vi "Run_2_of_5_Tests.vi"() -> ()   [LabVIEW 2019]
panel:
  out "Matrix":bool
  out "PID":bool
  out "Math Utils":bool
  out "Linear Filter":bool
  out "Linear System Loop":bool
  out "All Tests Finished":bool
  out "Holonomic Drive Ctrl":bool
  out "Linear Plant Inv FF":bool
  out "Numerical Jacobian":bool
  out "Merwe Scaled Sigma Pts":bool
  out "Numerical Integration":bool
  out "Median Filter":bool
  out "Linear System ID":bool
  out "Kalman filter":bool
  out "PID Input / Output":bool
  out "Linear Quadradtic Regulator":bool
  # "FORMAL TRAJECTORY / CONTROL LIBRARY TEST PROCEDURE"
  # "FUNCTION NOT\nIMPLEMENTED"
  # "Extended Kalman Filter"
  # "Mech Drive Kinematics"
  # "Mech Drive Odometry"
  # "Mech Drive Pose Est"
  # "FUNCTION NOT\nIMPLEMENTED"
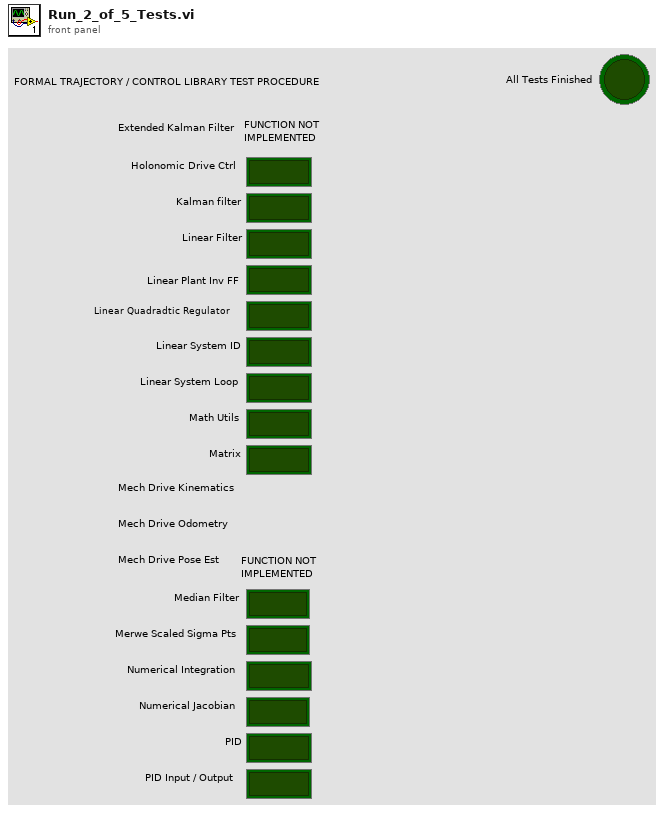
[diagram p1: front panel]
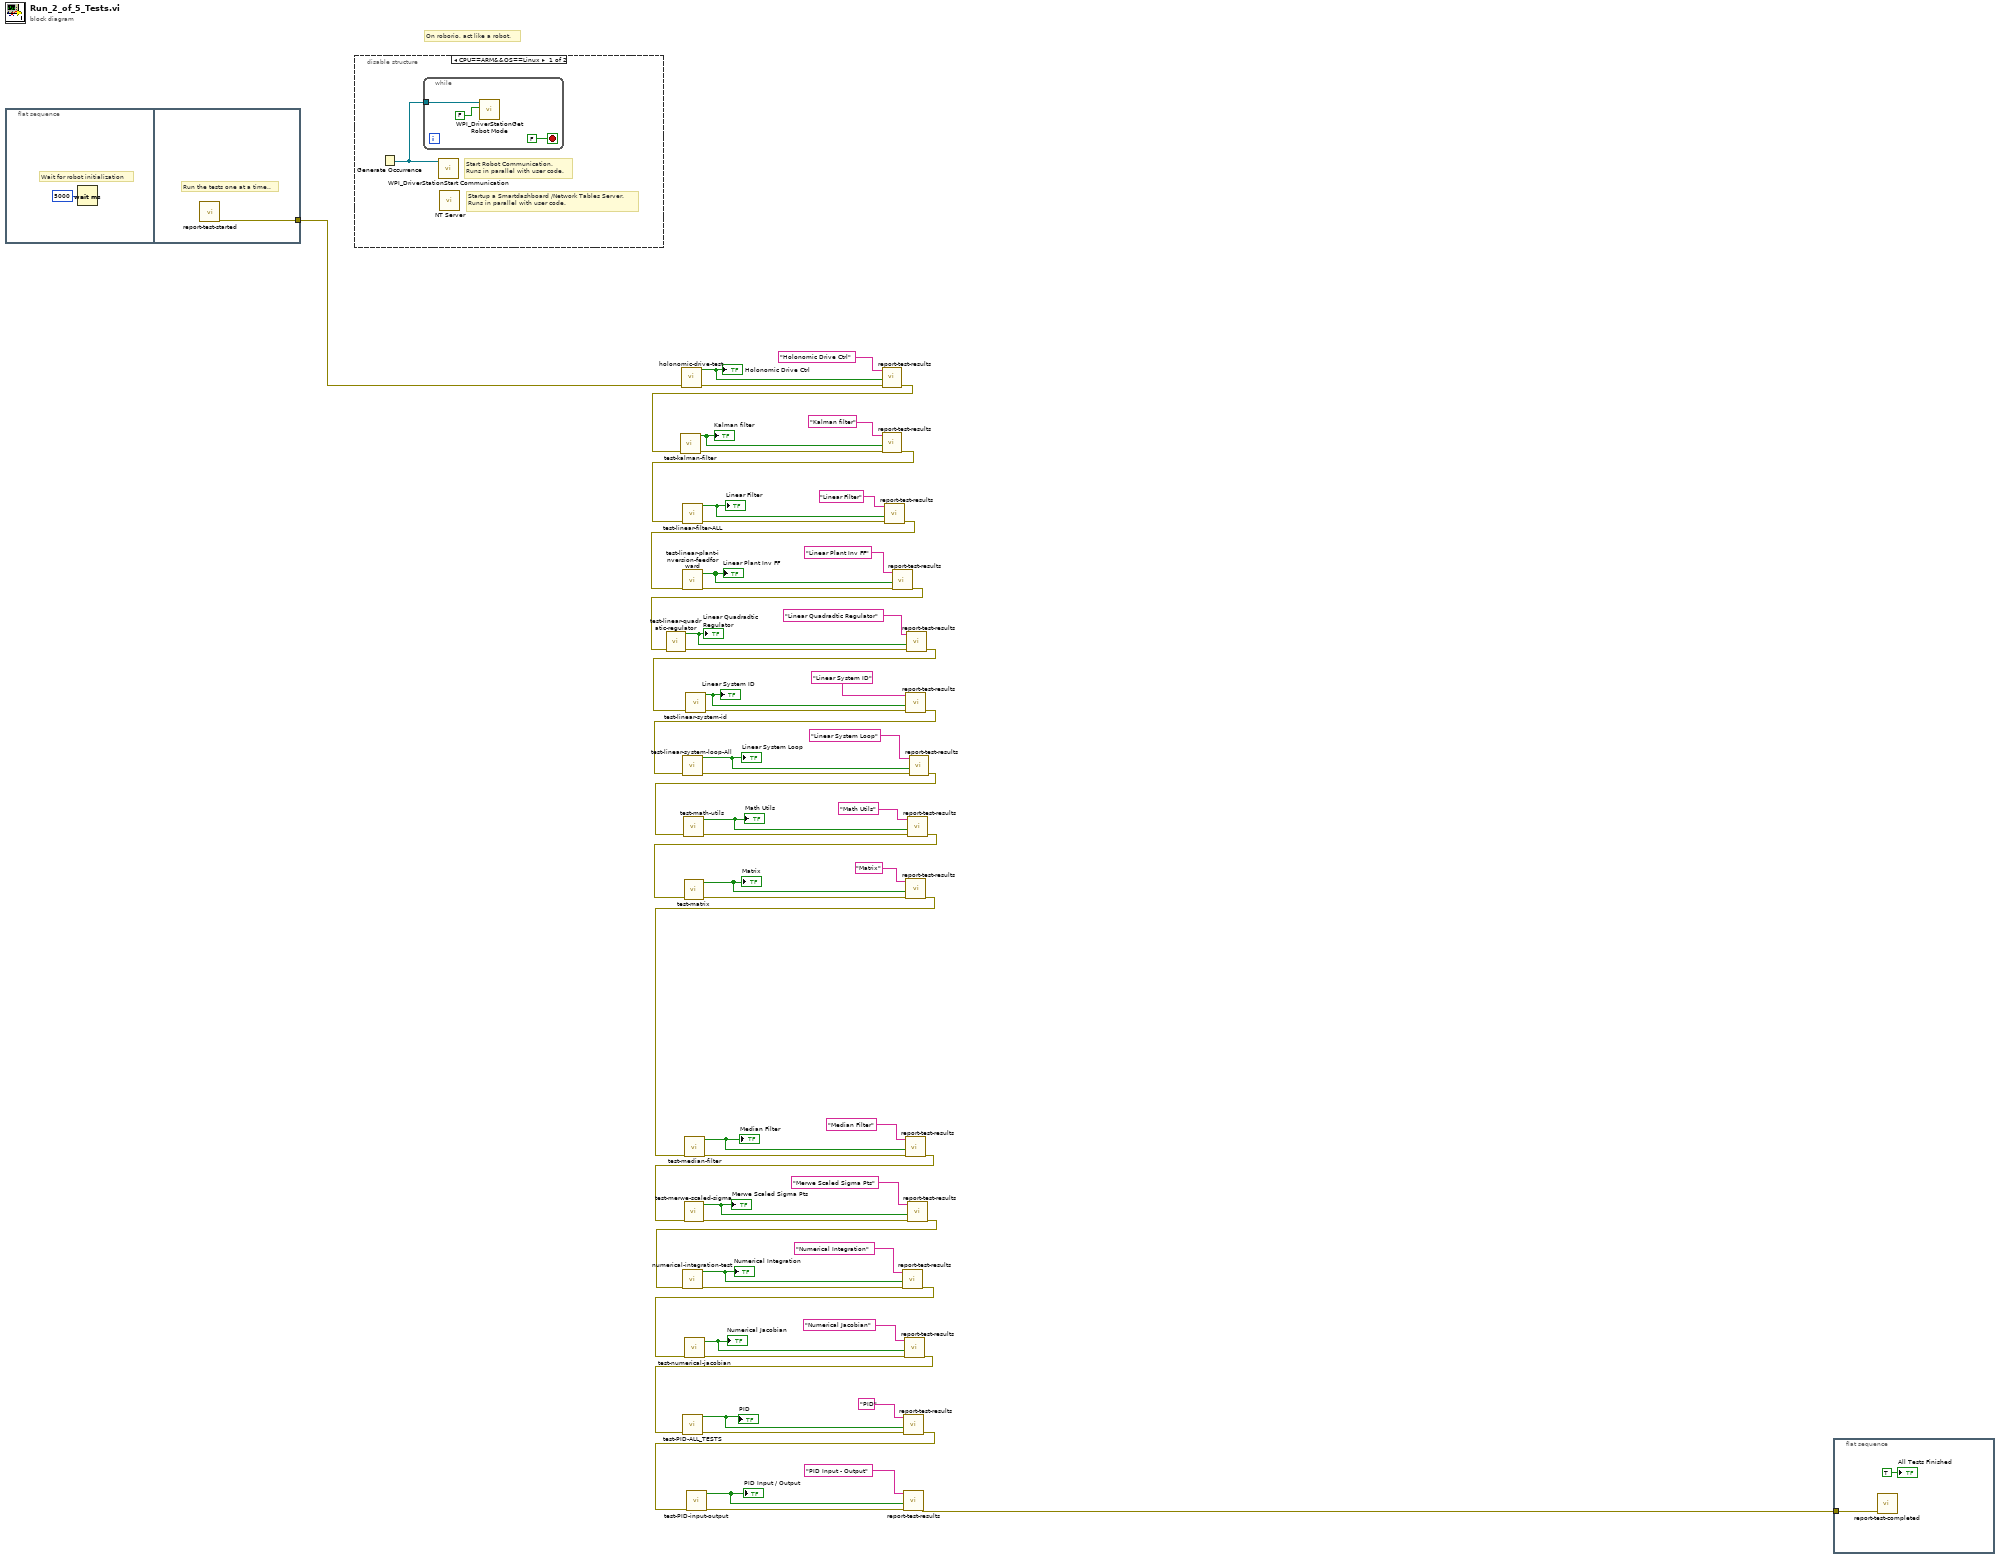
[diagram p0: block diagram]
diagram:
  # "On roborio, act like a robot."
  n1 = flat-sequence {
    tunnel: [w63] -> w1
    frame #0 {
      # "Wait for robot initialization"
      n2 = Wait (ms)(milliseconds to wait=u32 5000) -> ()  [unwired: 1 out]
    }
    frame #1 {
      # "Run the tests one at a time.."
      n3 = call "report-test-started.vi"() -> ("error out"=w63:errorcluster)  [unwired: 11 in]
    }
  }
  n4 = disable-structure shown="CPU==ARM&&OS==Linux" {
    frame condition #0 (active) {
      # "Startup a Smartdashboard /Network Tables Server.\nRuns in parallel with user code."
      # "Start Robot Communication.\nRuns in parallel with user code."
      n5 = Generate Occurrence() -> (w64:refnum<k4>)
      n6 = while {
        tunnel: w64 -> [w67]
        stop <- FALSE stop-if-true
        n7 = call <vilib>:"WPI_DriverStationGet Robot Mode.vi"("Finish"=FALSE, "DS Occurrence"=w67) -> ()  [unwired: 10 out]
      }
      n8 = call <vilib>:"WPI_DriverStationStart Communication.vi"("occurrence"=w64) -> ()  [unwired: 2 in, 9 out]
      n9 = call <vilib>:"NT Server.vi"() -> ()  [unwired: 12 in]
    }
    frame condition #1 {
    }
  }
  n10 = call "holonomic-drive-test.vi"("error in (no error)"=w1) -> ("error out"=w31:errorcluster, "ALL TESTS PASSED"=w59:bool)  [unwired: 9 in]
  "Holonomic Drive Ctrl" <- w59
  n11 = call "report-test-results.vi"("error in (no error)"=w31, "TestPassed"=w59, "Test Name"="Holonomic Drive Ctrl") -> ("error out"=w30:errorcluster)  [unwired: 8 in]
  n12 = call "test-kalman-filter.vi"("error in (no error)"=w30) -> ("error out"=w29:errorcluster, "ALL TESTS PASSED"=w58:bool)  [unwired: 9 in]
  "Kalman filter" <- w58
  n13 = call "report-test-results.vi"("error in (no error)"=w29, "TestPassed"=w58, "Test Name"="Kalman filter") -> ("error out"=w28:errorcluster)  [unwired: 8 in]
  n14 = call "test-linear-filter-ALL.vi"("error in (no error)"=w28) -> ("error out"=w26:errorcluster, "ALL TESTS GOOD"=w49:bool)  [unwired: 9 in]
  "Linear Filter" <- w49
  n15 = call "report-test-results.vi"("error in (no error)"=w26, "TestPassed"=w49, "Test Name"="Linear Filter") -> ("error out"=w25:errorcluster)  [unwired: 8 in]
  n16 = call "test-linear-plant-inversion-feedforward.vi"("error in (no error)"=w25) -> ("error out"=w24:errorcluster, "All Tests Passed"=w48:bool)  [unwired: 9 in]
  "Linear Plant Inv FF" <- w48
  n17 = call "report-test-results.vi"("error in (no error)"=w24, "TestPassed"=w48, "Test Name"="Linear Plant Inv FF") -> ("error out"=w23:errorcluster)  [unwired: 8 in]
  n18 = call "test-linear-quadratic-regulator.vi"("error in (no error)"=w23) -> ("error out"=w22:errorcluster, "ALL TESTS GOOD"=w47:bool)  [unwired: 9 in]
  "Linear Quadradtic Regulator" <- w47
  n19 = call "report-test-results.vi"("error in (no error)"=w22, "TestPassed"=w47, "Test Name"="Linear Quadradtic Regulator") -> ("error out"=w21:errorcluster)  [unwired: 8 in]
  n20 = call "test-linear-system-id.vi"("error in (no error)"=w21) -> ("error out"=w20:errorcluster, "All tests passed"=w46:bool)  [unwired: 9 in]
  "Linear System ID" <- w46
  n21 = call "report-test-results.vi"("error in (no error)"=w20, "TestPassed"=w46, "Test Name"="Linear System ID") -> ("error out"=w12:errorcluster)  [unwired: 8 in]
  n22 = call "test-linear-system-loop-All.vi"("error in (no error)"=w12) -> ("error out"=w13:errorcluster, "ALL TEsts Passed"=w45:bool)  [unwired: 9 in]
  "Linear System Loop" <- w45
  n23 = call "report-test-results.vi"("error in (no error)"=w13, "TestPassed"=w45, "Test Name"="Linear System Loop") -> ("error out"=w11:errorcluster)  [unwired: 8 in]
  n24 = call "test-math-utils.vi"("error in (no error)"=w11) -> ("error out"=w10:errorcluster, "ALL TESTS PASSED"=w44:bool)  [unwired: 9 in]
  "Math Utils" <- w44
  n25 = call "report-test-results.vi"("error in (no error)"=w10, "TestPassed"=w44, "Test Name"="Math Utils") -> ("error out"=w9:errorcluster)  [unwired: 8 in]
  n26 = call "test-matrix.vi"("error in (no error)"=w9) -> ("error out"=w14:errorcluster, "All Tests\nPassed"=w43:bool)  [unwired: 9 in]
  "Matrix" <- w43
  n27 = call "report-test-results.vi"("error in (no error)"=w14, "TestPassed"=w43, "Test Name"="Matrix") -> ("error out"=w8:errorcluster)  [unwired: 8 in]
  n28 = call "test-median-filter.vi"("error in (no error)"=w8) -> ("error out"=w15:errorcluster, "ALL TESTS PASSED"=w42:bool)  [unwired: 9 in]
  "Median Filter" <- w42
  n29 = call "report-test-results.vi"("error in (no error)"=w15, "TestPassed"=w42, "Test Name"="Median Filter") -> ("error out"=w7:errorcluster)  [unwired: 8 in]
  n30 = call "test-merwe-scaled-sigma.vi"("error in (no error)"=w7) -> ("error out"=w16:errorcluster, "All Tests Passed"=w32:bool)  [unwired: 9 in]
  "Merwe Scaled Sigma Pts" <- w32
  n31 = call "report-test-results.vi"("error in (no error)"=w16, "TestPassed"=w32, "Test Name"="Merwe Scaled Sigma Pts") -> ("error out"=w6:errorcluster)  [unwired: 8 in]
  n32 = call "numerical-integration-test.vi"("error in (no error)"=w6) -> ("error out"=w17:errorcluster, "All passed"=w33:bool)  [unwired: 9 in]
  "Numerical Integration" <- w33
  n33 = call "report-test-results.vi"("error in (no error)"=w17, "TestPassed"=w33, "Test Name"="Numerical Integration") -> ("error out"=w5:errorcluster)  [unwired: 8 in]
  n34 = call "test-numerical-jacobian.vi"("error in (no error)"=w5) -> ("error out"=w18:errorcluster, "ALL Tests Passed"=w34:bool)  [unwired: 9 in]
  "Numerical Jacobian" <- w34
  n35 = call "report-test-results.vi"("error in (no error)"=w18, "TestPassed"=w34, "Test Name"="Numerical Jacobian") -> ("error out"=w4:errorcluster)  [unwired: 8 in]
  n36 = call "test-PID-ALL_TESTS.vi"("error in (no error)"=w4) -> ("error out"=w19:errorcluster, "All Passed"=w35:bool)  [unwired: 9 in]
  "PID" <- w35
  n37 = call "report-test-results.vi"("error in (no error)"=w19, "TestPassed"=w35, "Test Name"="PID") -> ("error out"=w3:errorcluster)  [unwired: 8 in]
  n38 = call "test-PID-input-output.vi"("error in (no error)"=w3) -> ("error out"=w27:errorcluster, "All Passed"=w36:bool)  [unwired: 9 in]
  "PID Input / Output" <- w36
  n39 = call "report-test-results.vi"("error in (no error)"=w27, "TestPassed"=w36, "Test Name"="PID Input - Output") -> ("error out"=w2:errorcluster)  [unwired: 8 in]
  n40 = flat-sequence {
    tunnel: w2 -> [w68]
    frame #0 {
      n41 = call "report-test-completed.vi"("error in (no error)"=w68) -> ()  [unwired: 10 in, 1 out]
      "All Tests Finished" <- TRUE ("All Tests Finished")
    }
  }
